vi "Scanner Action-Status Stop Scan.vi"(8 "error in (no error)":errorcluster, 10 "Message Data":variant, 11 "Data Cluster in":T1={"Link"={"Connection"=enum."USB", "Host or IP address (TCP/IP)"="", "Port (Serial/USB)"="COM1"}, "VISA resource"="", "Writer Queue"=refnum, "Status"=FALSE}) -> (0 "error out":errorcluster, 3 "Data Cluster out":T1={"Link"={"Connection"=enum."USB", "Host or IP address (TCP/IP)"="", "Port (Serial/USB)"="COM1"}, "VISA resource"="", "Writer Queue"=refnum, "Status"=FALSE})   [LabVIEW 2020, in "Hiden Scanner.lvlib"]
uses:
  Hiden Scanner.lvlib
  Scanner Hardware Configuration.ctl
  support/Message Queue/Message Cluster.ctl
  support/HW Message Cluster.ctl
  support/Message Queue/Message Queue.lvlib
  <instrlib>/Hiden/Hiden MS.lvlib
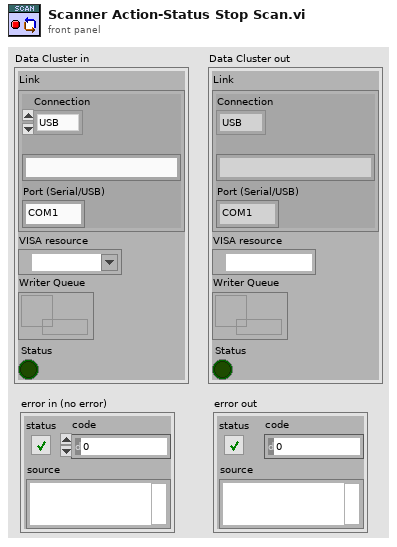
[diagram p1: front panel]
types:
  T1 = typedef "Hiden Scanner.lvlib/Scanner Hardware Configuration.ctl" = cluster{"Link":cluster{"Connection":enum16{"Serial", "TCP/IP", "USB"}, "Host or IP address (TCP/IP)":string, "Port (Serial/USB)":string}, "VISA resource":refnum<visa-resource-name>, "Writer Queue":refnum<queue>, "Status":bool}
  T2 = typedef "Message Queue.lvlib/HW Message Cluster.ctl" = cluster{"Writer Queue":refnum<queue>, "Writer Data":T3}
  T3 = typedef "Message Queue.lvlib/Message Cluster.ctl" = cluster{"Message":string, "Message Data":variant}
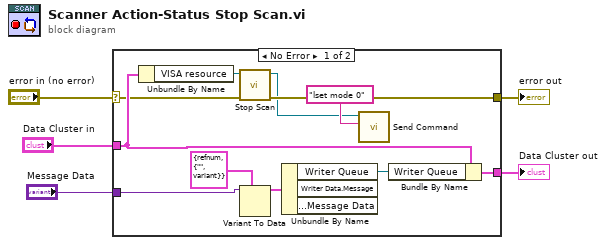
[diagram p0: block diagram]
diagram:
  n1 = case shown="No Error" "error in (no error)" {
    selector: "error in (no error)" -> [w9 w17]
    tunnel: "Message Data" -> [w13 _]
    tunnel: [w16 w18] -> w4
    tunnel: "Data Cluster in" -> [w11 w18]
    tunnel: [w8 w17] -> w2
    frame No Error {
      n2 = Unbundle By Name(w11) -> ("VISA resource"=w10:refnum<visa-resource-name>)
      n3 = call <instrlib>:"Stop Scan.vi"("error in (no error)"=w9, "Connection"=w10) -> ("error out"=w8:errorcluster, "Connection (dup)"=w6:refnum<visa-resource-name>)  [unwired: 8 in]
      n4 = Variant To Data(type=T2 {"Writer Queue"=refnum, "Writer Data"={"Message"="", "Message Data"=variant}}, Variant=w13) -> (data=w15:T2)  [unwired: 1 in, 1 out]
      n5 = Unbundle By Name(w15) -> ("Writer Queue"=w12:refnum<queue>)  [unwired: 2 out]
      n6 = call <instrlib>:"Send Command.vi"("Command"="lset mode 0", "Connection"=w6) -> ()  [unwired: 7 in, 3 out]
      n7 = Bundle By Name(cluster=w11, "Writer Queue"=w12) -> (w16:T1)
    }
    frame Error {
    }
  }
  "Data Cluster out" <- w4
  "error out" <- w2
